vi "Write.vi"(10 "Waveform":waveform(dbl), 11 "Waveform in":refnum<class "Waveform.lvclass">) -> (3 "Waveform out":refnum<class "Waveform.lvclass">)   [LabVIEW 2020, in "Data.lvlib" / "Waveform.lvclass"]
doc: "Write Waveform."
uses:
  Waveform.lvclass
  Waveform.lvclass/Waveform.ctl
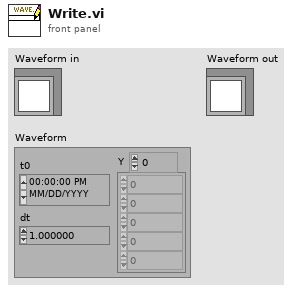
[diagram p1: front panel]
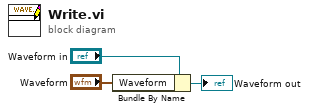
[diagram p0: block diagram]
diagram:
  n1 = Bundle By Name(cluster="Waveform in", "Waveform"="Waveform") -> (→"Waveform out":refnum<class "Waveform.lvclass">)
